vi "Position Mean - Plugin Main.vi"(11 "Shared Data from EMA":T2={"Impulse Positions"=[], "Parameter Impuls Series"=[], "Data File"={"Data Channels"=[], "Sample Rate"=0, "Channel List"=[]}, "desacc "={"Threshold 1 [Acc]"=7000.0, "Threshold 2 [% of TH1]"=60, "tolerance"=3, "Search WD "=0.1, " always use TH2"=FALSE, "Range"=2.0, "Max time"=120.0, "Min time"=20.0, "Velocity Threshold"=150}, "Experiment Parameters 2"={"Subject"="", "Strain"="", "Rotation plane"="", "Experimenter"="", "Trial"=0.0, "Time"=0.0}} {"Parameter Impuls Series"."Gain" format="%.1f"; "Parameter Impuls Series"."Offset" format="%.1f"}) -> (3 "Shared Data from EMA 2":T2={"Impulse Positions"=[], "Parameter Impuls Series"=[], "Data File"={"Data Channels"=[], "Sample Rate"=0, "Channel List"=[]}, "desacc "={"Threshold 1 [Acc]"=7000.0, "Threshold 2 [% of TH1]"=60, "tolerance"=3, "Search WD "=0.1, " always use TH2"=FALSE, "Range"=2.0, "Max time"=120.0, "Min time"=20.0, "Velocity Threshold"=150}, "Experiment Parameters 2"={"Subject"="", "Strain"="", "Rotation plane"="", "Experimenter"="", "Trial"=0.0, "Time"=0.0}} {"Parameter Impuls Series"."Gain" format="%.1f"; "Parameter Impuls Series"."Offset" format="%.1f"})   [LabVIEW 2013]
uses:
  Plugin Shared Data.ctl
  core/type-defs/TD_Impulse Parameter.ctl
  res/controls/impuls graph/impuls graph.xctl
  <vilib>/Analysis/baseanly.llb/Mean (DBL).vi
  comm/impulse/impulse functions.lvlib
  <vilib>/Analysis/NI_AALBase.lvlib
  <vilib>/ptbypt/NI_PtbyPt.lvlib
  core/core.lvlib
  plugin data.lvlib
panel:
  out "Waveform Graph":dbl[][](graph)
  out "Impulse Plot":T1(xcontrol)
  out "Waveform Graph 2":dbl[][](graph)
  in  "Delete trace":bool
  in  "Button toClipboard":bool
  in  "Button Save":bool
  in  "Table":string[][](table)
  out "K":dbl format="%#.3e"
  out "Distance":dbl format="%#.2g"
  out "Distance SD":dbl format="%#.2g"
  in  "Button Calculate":bool
  out "K SD":dbl format="%#.2g"
  in  "Parameter Impuls Series":T3=[{"Color"=4652800, "Visible"=TRUE, "Channel"=5, "Invert"=FALSE, "Desaccade"=FALSE, "Offset"=0.0, "Gain"=1.0}, {"Color"=16860, "Visible"=TRUE, "Channel"=13, "Invert"=FALSE, "Desaccade"=FALSE, "Offset"=0.0, "Gain"=1.0}, {"Color"=16711680, "Visible"=TRUE, "Channel"=21, "Invert"=FALSE, "Desaccade"=FALSE, "Offset"=0.0, "Gain"=1.0}] {"Gain" format="%.1f"; "Offset" format="%.1f"}
  in  "Impulse Direction":bool
  in  "Mean and STD":bool
  in  "Delete trace 2":bool
  in  "Stop Button":bool
  # "Offset         Gain    Inv                    Channel                         Col   Vis   Sac"
  # "Pos"
  # "Neg"
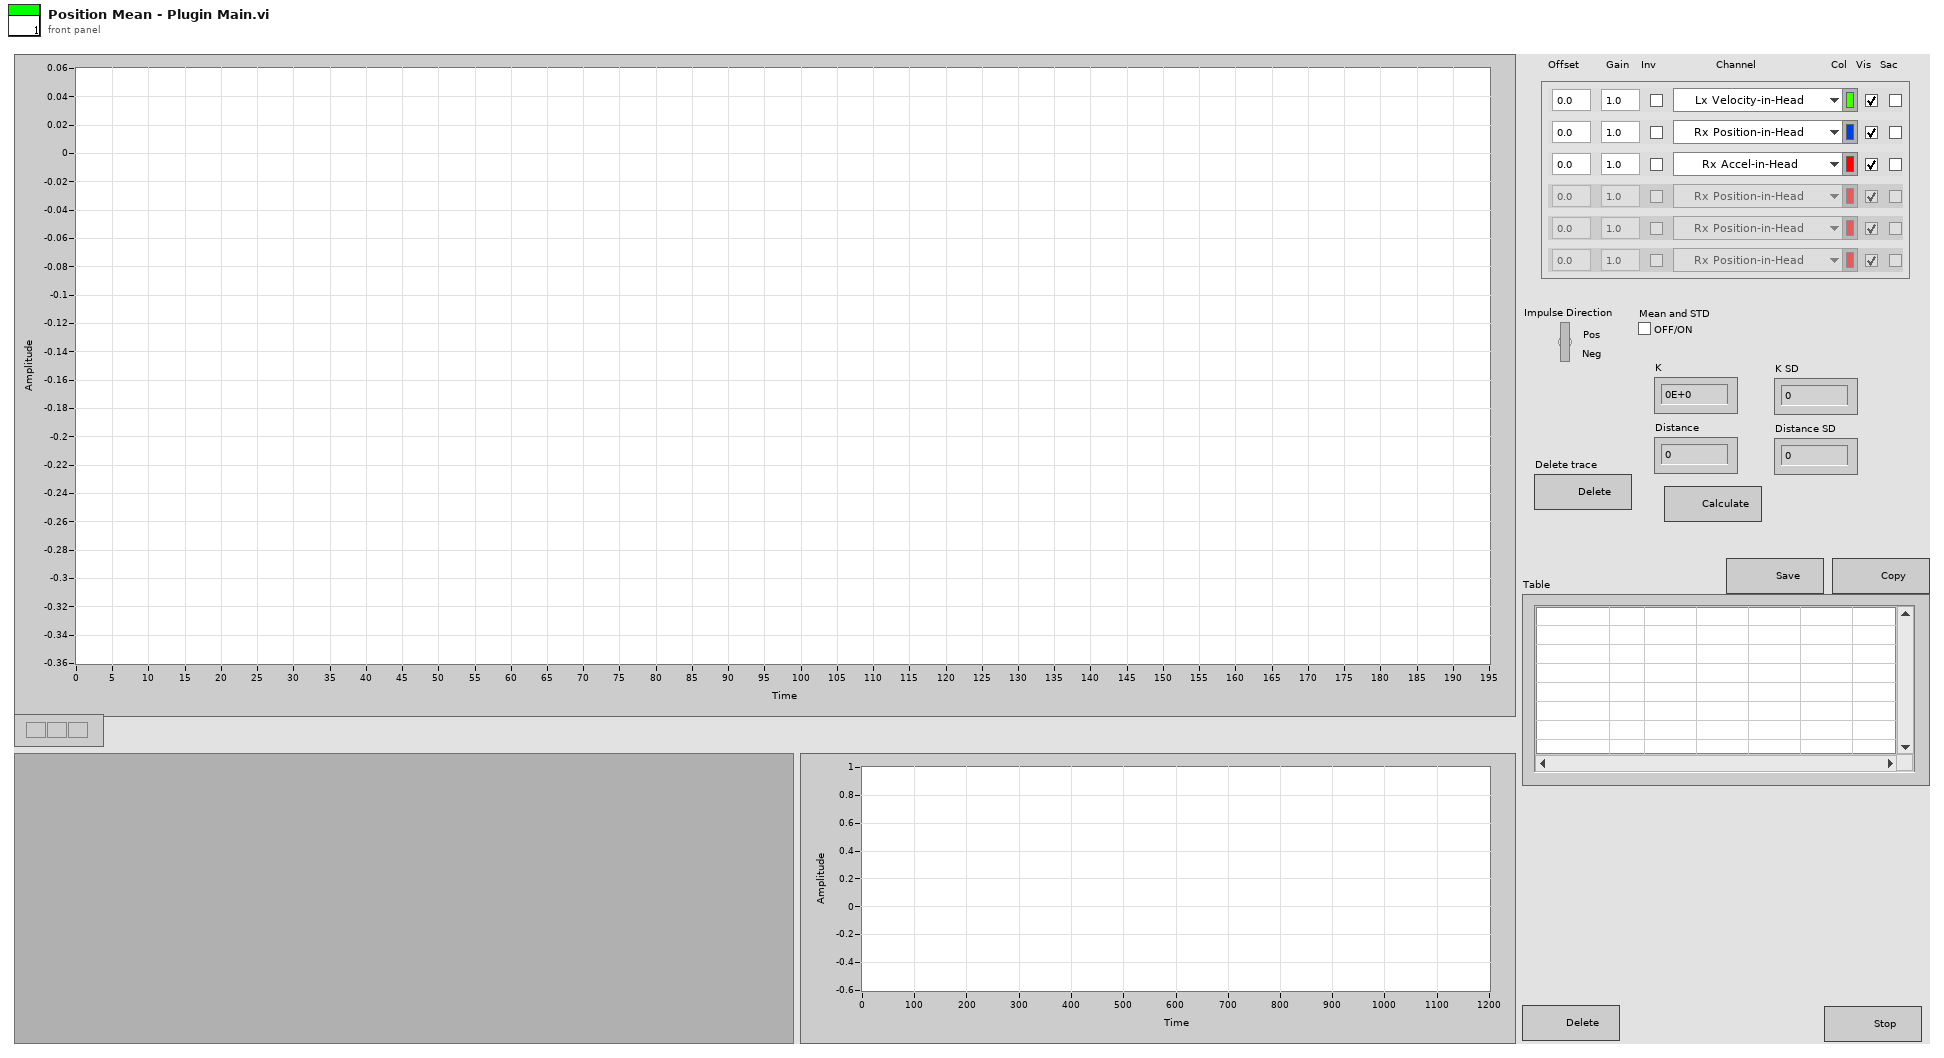
[diagram p1: front panel]
types:
  T1 = cluster{"Data":dbl[][], "Colour":u32, "Channel Name":string, "Sample Rate":dbl, "Visible":bool}[]
  T2 = typedef "plugin data.lvlib/Plugin Shared Data.ctl" = cluster{"Impulse Positions":cluster{"Start":i32, "End":i32, "Impulse Plane":enum16{"Other", "Yaw", "Pitch", "Roll", "LARP", "RALP"}, "Impulse Direction +ve?":bool, "Time offset":i32, "Amplitude offset":dbl}[], "Parameter Impuls Series":T3, "Data File":cluster{"Data Channels":dbl[][], "Sample Rate":i32, "Channel List":string[]}, "desacc ":cluster{"Threshold 1 [Acc]":dbl, "Threshold 2 [% of TH1]":i32, "tolerance":i32, "Search WD ":dbl, " always use TH2":bool, "Range":dbl, "Max time":dbl, "Min time":dbl, "Velocity Threshold":i32}, "Experiment Parameters 2":cluster{"Subject":string, "Strain":string, "Rotation plane":string, "Experimenter":string, "Trial":dbl, "Time":dbl}}
  T3 = typedef "core.lvlib/TD_Impulse Parameter.ctl" = cluster{"Color":u32, "Visible":bool, "Channel":u16, "Invert":bool, "Desaccade":bool, "Offset":dbl, "Gain":dbl}[]
  T4 = cluster{"Example Data":bool, "Impuls Data":cluster{"Data":dbl[][], "Colour":u32, "Channel Name":string, "Sample Rate":dbl, "Visible":bool}[], "K":dbl[], "cum pos data":dbl[][]}
  T5 = enum16{"Other", "Yaw", "Pitch", "Roll", "LARP", "RALP"}
  T6 = cluster{"Data Channels":dbl[][], "Sample Rate":i32, "Channel List":string[]}
  T7 = cluster{"Start":i32, "End":i32, "Impulse Plane":enum16{"Other", "Yaw", "Pitch", "Roll", "LARP", "RALP"}, "Impulse Direction +ve?":bool, "Time offset":i32, "Amplitude offset":dbl}[]
  T8 = cluster{"Threshold 1 [Acc]":dbl, "Threshold 2 [% of TH1]":i32, "tolerance":i32, "Search WD ":dbl, " always use TH2":bool, "Range":dbl, "Max time":dbl, "Min time":dbl, "Velocity Threshold":i32}
  T9 = typedef "LVCursorListTypeDef.ctl" = cluster{"Name":string, "Color":u32, "Style":u8, "Point Style":u8, "Name Visible":bool, "Allow Drag":bool, "Cursor Mode":u32, "Plot":i32, "Index":i32, "Position":cluster{"X":dbl, "Y":dbl}, "X Scale":u32, "Y Scale":u32, "Watch Plots":i32[], "Watch All Plots":bool, "Plot Area":i32, "Label Offset":cluster{"X":dbl, "Y":dbl}}[]
  T10 = cluster{"Name":string, "Color":u32, "Style":u8, "Point Style":u8, "Name Visible":bool, "Allow Drag":bool, "Cursor Mode":u32, "Plot":i32, "Index":i32, "Position":cluster{"X":dbl, "Y":dbl}, "X Scale":u32, "Y Scale":u32, "Watch Plots":i32[], "Watch All Plots":bool, "Plot Area":i32, "Label Offset":cluster{"X":dbl, "Y":dbl}}
  T11 = cluster{"Data":dbl[][], "Colour":u32, "Channel Name":string, "Sample Rate":dbl, "Visible":bool}
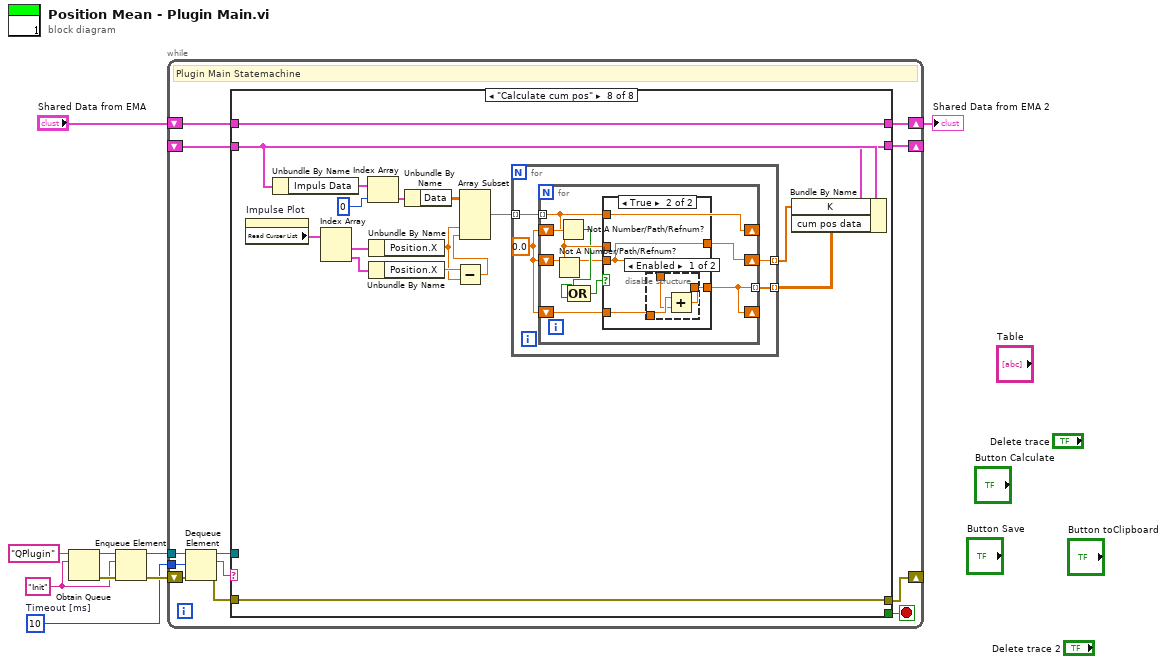
[diagram p0: block diagram]
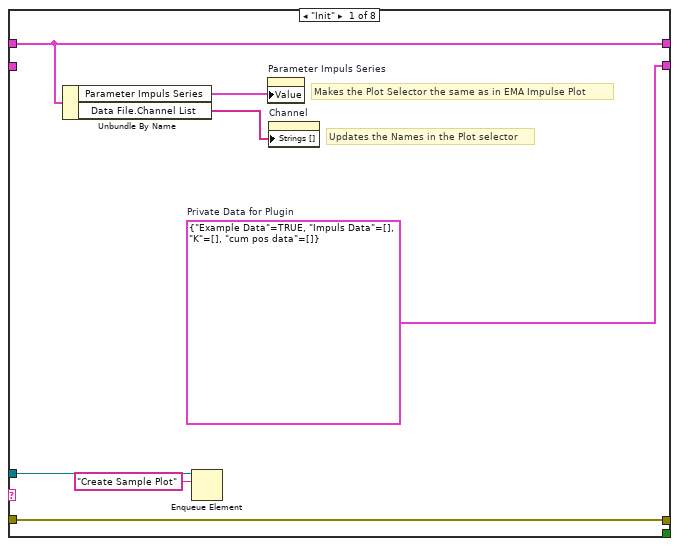
[diagram p2: hidden frame]
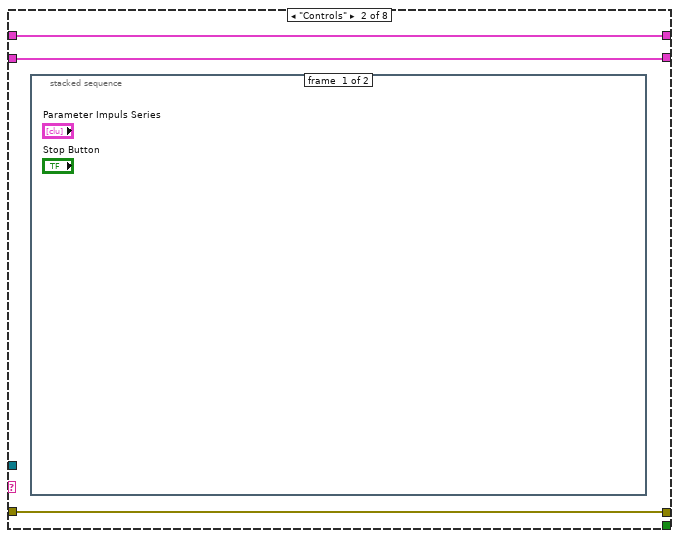
[diagram p3: hidden frame]
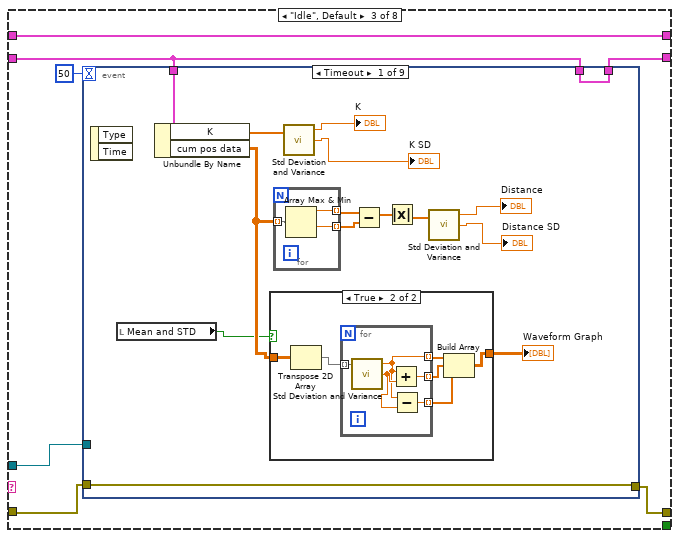
[diagram p5: hidden frame]
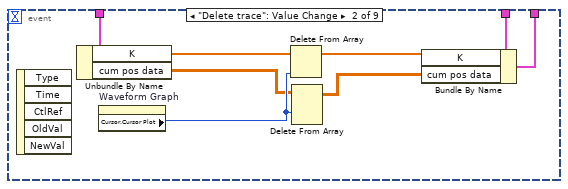
[diagram p7: hidden frame]
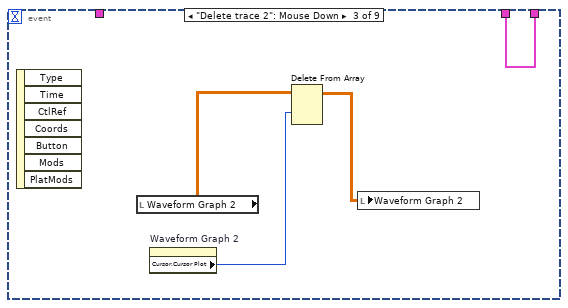
[diagram p8: hidden frame]
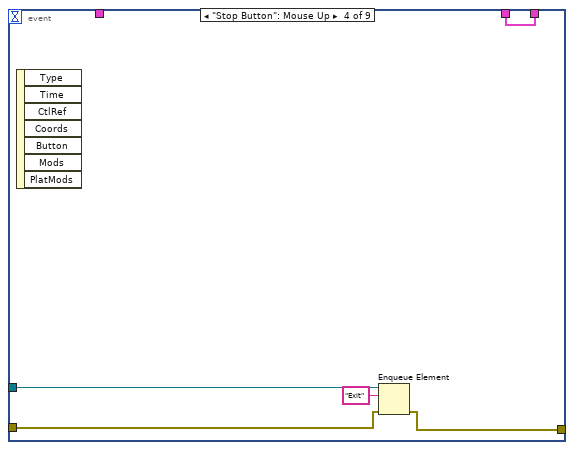
[diagram p9: hidden frame]
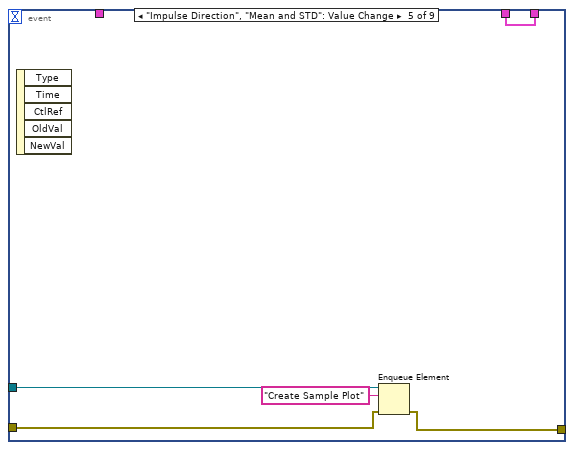
[diagram p10: hidden frame]
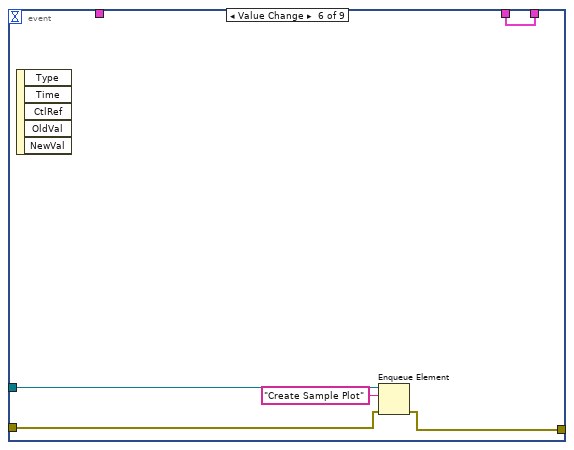
[diagram p11: hidden frame]
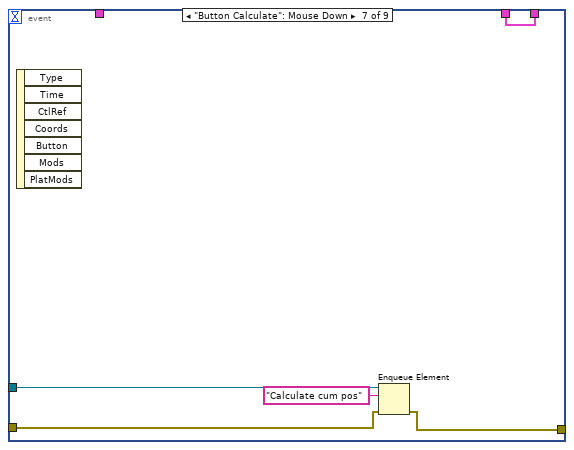
[diagram p12: hidden frame]
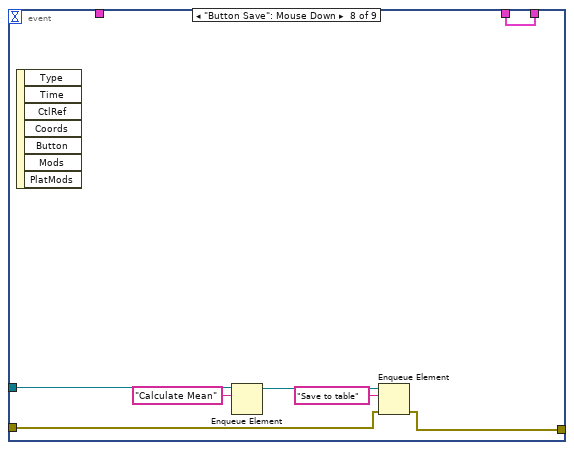
[diagram p13: hidden frame]
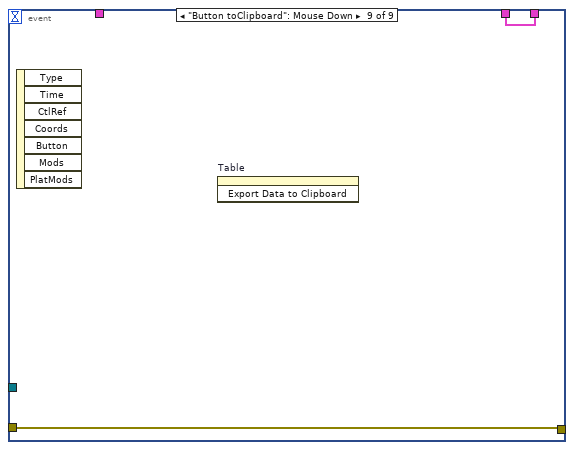
[diagram p14: hidden frame]
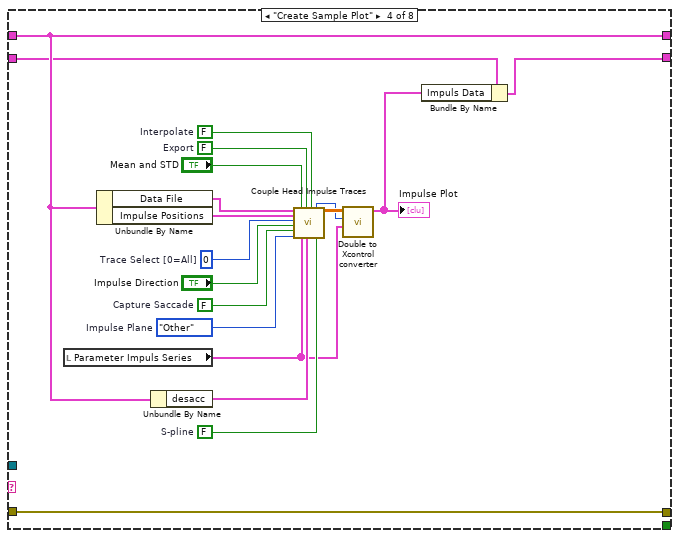
[diagram p15: hidden frame]
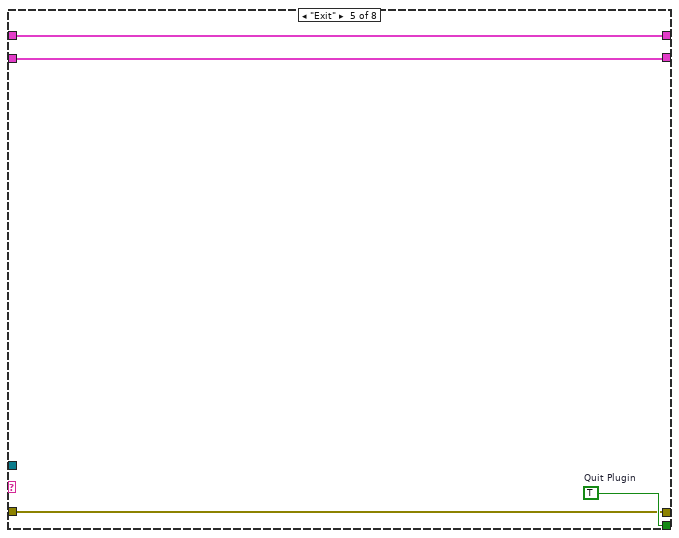
[diagram p16: hidden frame]
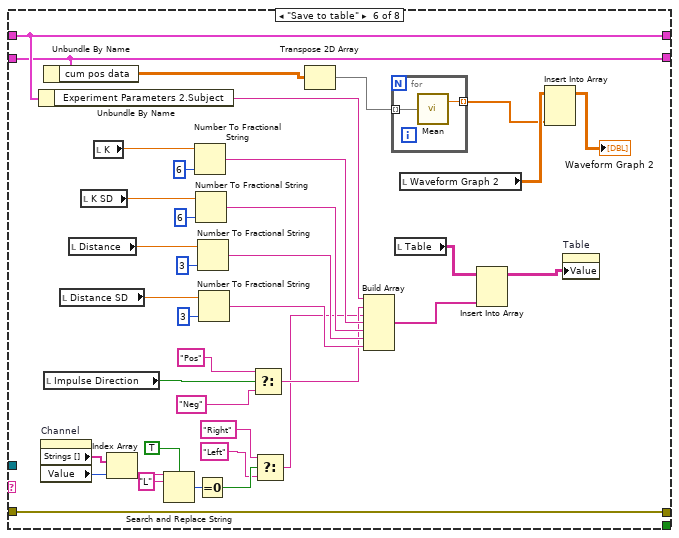
[diagram p17: hidden frame]
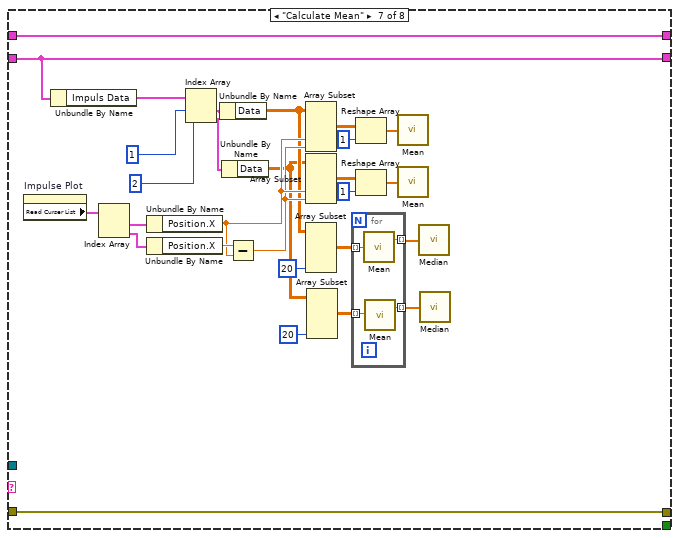
[diagram p18: hidden frame]
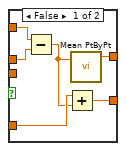
[diagram p19: hidden frame]
diagram:
  w3 = 10  # Timeout [ms]
  w7 = "Init"
  n1 = Obtain Queue(name (unnamed)="QPlugin", element data type=w7) -> (queue out=w8:refnum<queue>, error out=w9:errorcluster)  [unwired: 3 in, 1 out]
  n2 = Enqueue Element(queue=w8, element=w7, error in (no error)=w9) -> (queue out=w5:refnum<queue>, error out=w4:errorcluster)  [unwired: 1 in, 1 out]
  n3 = while {
    tunnel: w5 -> [w20]
    tunnel: w3 -> [w18]
    shift-right: [w14] -> _
    shift-left: w4 -> [w19]
    shift-right: [w13] -> _
    shift-left: _ -> [w12]
    shift-right: [w10] -> w1
    shift-left: "Shared Data from EMA" -> [w11]
    stop <- w21 stop-if-true
    # "Plugin Main Statemachine"
    n4 = Dequeue Element(queue=w20, timeout in ms (-1)=w18, error in (no error)=w19) -> (queue out=w17:refnum<queue>, element=w16:string, error out=w15:errorcluster)  [unwired: 1 out]
    n5 = case shown="\"Calculate cum pos\"" w16 {
      tunnel: [_ _ _ _ w132 _ _ _] -> w21
      tunnel: w17 -> [w26 _ w37 _ _ _ _ _]
      tunnel: w15 -> [w27 w29 w36 w128 w131 w170 w200 w221]
      tunnel: [w27 w29 w35 w128 w131 w170 w200 w221] -> w14
      tunnel: [w28 w30 w32 w111 w130 w138 w198 w207] -> w13
      tunnel: w12 -> [_ w30 w33 w112 w130 w138 w198 w208]
      tunnel: w11 -> [w24 w31 w38 w118 w129 w169 w199 w220]
      tunnel: [w24 w31 w38 w118 w129 w169 w199 w220] -> w10
      frame "Init" {
        w28 = T4 {"Example Data"=TRUE, "Impuls Data"=[], "K"=[], "cum pos data"=[]}  # Private Data for Plugin
        # "Makes the Plot Selector the same as in EMA Impulse Plot"
        # "Updates the Names in the Plot selector"
        n6 = Unbundle By Name(w24) -> ("Parameter Impuls Series"=w23:T3, "Data File.Channel List"=w22:string[])
        n7 = Enqueue Element(queue=w26, element="Create Sample Plot") -> ()  [unwired: 2 in, 3 out]
        n8 = property on="Parameter Impuls Series" class="Arr (strict)"("Value"=w23) -> ()  [unwired: 2 in, 2 out]
        n9 = property on="Channel" class="Ring (strict)"("Strings []"=w22) -> ()  [unwired: 2 in, 2 out]
      }
      frame "Controls" {
        n10 = stacked-sequence {
          frame #0 {
          }
          frame #1 {
          }
        }
      }
      frame "Idle", Default {
        n11 = event shown="[0] Timeout" {
          selector: _ -> [_ _ _ _ _ _ _ _ _]
          dyn-events: _ -> [_ _ _ _ _ _ _ _ _]
          timeout: 50 -> [_ _ _ _ _ _ _ _ _]
          tunnel: w37 -> [_ _ _ w85 w90 w95 w100 w104 _]
          tunnel: w36 -> [w53 _ _ w83 w88 w93 w98 w106 w109]
          tunnel: [w53 _ _ w82 w87 w92 w97 w105 w109] -> w35
          tunnel: w33 -> [w52 w76 _ _ _ _ _ _ _]
          tunnel: w33 -> [w51 w74 w80 w81 w86 w91 w96 w101 w108]
          tunnel: [w51 w71 w80 w81 w86 w91 w96 w101 w108] -> w32
          event Timeout {
            n12 = event-data() -> ()  [unwired: 1 in, 2 out]
            n13 = local read "Mean and STD"() -> (w45:bool)
            n14 = Unbundle By Name(w52) -> ("K"=w39:dbl[], "cum pos data"=w47:dbl[][])
            n15 = case shown="True" w45 {
              tunnel: w47 -> [w54 w60]
              tunnel: [w54 w57] -> w46
              frame False {
              }
              frame True {
                n16 = Transpose 2D Array(2D array=w60) -> (transposed array=w59:dbl[][])
                n17 = for {
                  tunnel: w59 -> [w65] mode=indexing
                  tunnel: [w61] -> w58 mode=indexing
                  tunnel: [w63] -> w56 mode=indexing
                  tunnel: [w62] -> w55 mode=indexing
                  n18 = call <vilib>:"Std Deviation and Variance.vi"("X"=w65) -> ("mean"=w61:dbl, "standard deviation"=w64:dbl)  [unwired: 1 in, 1 out]
                  n19 = Add(x=w61, y=w64) -> (x+y=w63:dbl)
                  n20 = Subtract(x=w61, y=w64) -> (x-y=w62:dbl)
                }
                n21 = Build Array(w58, w56, w55) -> (w57:dbl[][])
              }
            }
            "Waveform Graph" <- w46
            n22 = for {
              tunnel: w47 -> [w68] mode=indexing
              tunnel: [w67] -> w50 mode=indexing
              tunnel: [w66] -> w49 mode=indexing
              n23 = Array Max & Min(array=w68) -> (max value=w67:dbl, min value=w66:dbl)  [unwired: 2 out]
            }
            n24 = call <vilib>:"Std Deviation and Variance.vi"("X"=w39) -> ("mean"=→"K":dbl, "standard deviation"=→"K SD":dbl)  [unwired: 1 in, 1 out]
            n25 = Subtract(x=w50, y=w49) -> (x-y=w48:dbl[])
            n26 = Absolute Value(x=w48) -> (abs(x)=w44:dbl[])
            n27 = call <vilib>:"Std Deviation and Variance.vi"("X"=w44) -> ("mean"=→"Distance":dbl, "standard deviation"=→"Distance SD":dbl)  [unwired: 1 in, 1 out]
          }
          event "Delete trace": Value Change {
            n28 = event-data() -> ()  [unwired: 1 in, 5 out]
            n29 = Unbundle By Name(w76) -> ("K"=w75:dbl[], "cum pos data"=w69:dbl[][])
            n30 = property on="Waveform Graph" class="WFGraph (strict)"() -> ("Cursor.Cursor Plot"=w70:i32)  [unwired: 2 in, 2 out]
            n31 = Delete From Array(array=w75, index=w70) -> (array with subset deleted=w73:dbl[])  [unwired: 1 in, 1 out]
            n32 = Delete From Array(array=w69, index (row)=w70) -> (array with subset deleted=w72:dbl[][])  [unwired: 2 in, 1 out]
            n33 = Bundle By Name(cluster=w74, "K"=w73, "cum pos data"=w72) -> (w71:T4)
          }
          event "Delete trace 2": Mouse Down {
            n34 = event-data() -> ()  [unwired: 1 in, 7 out]
            n35 = local read "Waveform Graph 2"() -> (w79:dbl[][])
            n36 = property on="Waveform Graph 2" class="WFGraph (strict)"() -> ("Cursor.Cursor Plot"=w77:i32)  [unwired: 2 in, 2 out]
            n37 = Delete From Array(array=w79, index (row)=w77) -> (array with subset deleted=w78:dbl[][])  [unwired: 2 in, 1 out]
            n38 = local write "Waveform Graph 2"(w78) -> ()
          }
          event "Stop Button": Mouse Up {
            n39 = event-data() -> ()  [unwired: 1 in, 7 out]
            n40 = Enqueue Element(queue=w85, element="Exit", error in (no error)=w83) -> (error out=w82:errorcluster)  [unwired: 1 in, 2 out]
          }
          event "Impulse Direction", "Mean and STD": Value Change {
            n41 = event-data() -> ()  [unwired: 1 in, 5 out]
            n42 = Enqueue Element(queue=w90, element="Create Sample Plot", error in (no error)=w88) -> (error out=w87:errorcluster)  [unwired: 1 in, 2 out]
          }
          event Value Change {
            n43 = event-data() -> ()  [unwired: 1 in, 5 out]
            n44 = Enqueue Element(queue=w95, element="Create Sample Plot", error in (no error)=w93) -> (error out=w92:errorcluster)  [unwired: 1 in, 2 out]
          }
          event "Button Calculate": Mouse Down {
            n45 = event-data() -> ()  [unwired: 1 in, 7 out]
            n46 = Enqueue Element(queue=w100, element="Calculate cum pos", error in (no error)=w98) -> (error out=w97:errorcluster)  [unwired: 1 in, 2 out]
          }
          event "Button Save": Mouse Down {
            n47 = event-data() -> ()  [unwired: 1 in, 7 out]
            n48 = Enqueue Element(queue=w104, element="Calculate Mean") -> (queue out=w103:refnum<queue>)  [unwired: 2 in, 2 out]
            n49 = Enqueue Element(queue=w103, element="Save to table", error in (no error)=w106) -> (error out=w105:errorcluster)  [unwired: 1 in, 2 out]
          }
          event "Button toClipboard": Mouse Down {
            n50 = event-data() -> ()  [unwired: 1 in, 7 out]
            n51 = invoke on="Table" class="Tbl (strict)" method="Export Data to Clipboard"() -> ()  [unwired: 3 in, 3 out]
          }
        }
      }
      frame "Create Sample Plot" {
        w116 = FALSE  # S-pline
        w119 = FALSE  # Interpolate
        w120 = FALSE  # Export
        w122 = T5."Other"  # Impulse Plane
        w123 = FALSE  # Capture Saccade
        w125 = 0  # Trace Select [0=All]
        n52 = local read "Parameter Impuls Series"() -> (w113:T3)
        n53 = Unbundle By Name(w118) -> ("Data File"=w126:T6, "Impulse Positions"=w127:T7)
        n54 = Unbundle By Name(w118) -> ("desacc"=w117:T8)
        n55 = call "Couple Head Impulse Traces.vi"("Data Input"=w126, "Impulse Positions"=w127, "Trace Select"=w125, "Impulse Direction +ve?"="Impulse Direction", "Capture Saccade"=w123, "Impulse Plane"=w122, "Mean and STD"="Mean and STD", "Plot Selection 2"=w113, "Export"=w120, "desacc"=w117, "Interpolate"=w119, "S-pline"=w116) -> ("No Impulses"=w114:i32, "Impulses"=w115:dbl[][])  [unwired: 4 in, 2 out]
        n56 = call "Double to Xcontrol converter.vi"("Parameter Impuls Series"=w113, "No Impulses"=w114, "Impulses"=w115) -> ("Array"=w110:T1)  [unwired: 8 in]
        "Impulse Plot" <- w110
        n57 = Bundle By Name(cluster=w112, "Impuls Data"=w110) -> (w111:T4)
      }
      frame "Exit" {
        w132 = TRUE  # Quit Plugin
      }
      frame "Save to table" {
        n58 = Unbundle By Name(w169) -> ("Experiment Parameters 2.Subject"=w167:string)
        n59 = property on="Channel" class="Ring (strict)"() -> ("Strings []"=w148:string[], "Value"=w147:u16)  [unwired: 2 in, 2 out]
        n60 = Unbundle By Name(w138) -> ("cum pos data"=w136:dbl[][])
        n61 = local read "Impulse Direction"() -> (w152:bool)
        n62 = local read "Distance SD"() -> (w157:dbl)
        n63 = local read "Distance"() -> (w158:dbl)
        n64 = local read "K SD"() -> (w159:dbl)
        n65 = local read "K"() -> (w166:dbl)
        n66 = Index Array(array=w148, index=w147) -> (element=w146:string)
        n67 = Search and Replace String(case sensitive?=TRUE ("ignore case? (F)"), input string=w146, search string="L") -> (number of replacements=w143:i32)  [unwired: 5 in, 3 out]
        n68 = Number To Fractional String(number=w166, precision (6)=i16 6) -> (F-format string=w156:string)  [unwired: 2 in]
        n69 = Number To Fractional String(number=w159, precision (6)=i16 6) -> (F-format string=w155:string)  [unwired: 2 in]
        n70 = Equal To 0?(x=w143) -> (x = 0?=w142:bool)
        n71 = Number To Fractional String(number=w158, precision (6)=i16 3) -> (F-format string=w154:string)  [unwired: 2 in]
        n72 = Number To Fractional String(number=w157, precision (6)=i16 3) -> (F-format string=w153:string)  [unwired: 2 in]
        n73 = Select(t="Pos", s=w152, f="Neg") -> (s? t:f=w151:string)
        n74 = Select(t="Right", s=w142, f="Left") -> (s? t:f=w139:string)
        n75 = Transpose 2D Array(2D array=w136) -> (transposed array=w137:dbl[][])
        n76 = Build Array(w167, w151, w139, w156, w155, w154, w153) -> (w164:string[])
        n77 = for {
          tunnel: w137 -> [w172] mode=indexing
          tunnel: [w171] -> w134 mode=indexing
          n78 = call-poly <vilib>:"Mean.vi"("X"=w172) -> ("mean"=w171:dbl)  [unwired: 1 out]
        }
        n79 = local read "Table"() -> (w168:string[][])
        n80 = local read "Waveform Graph 2"() -> (w135:dbl[][])
        n81 = Insert Into Array(array=w168, new element=w164) -> (w163:string[][])  [unwired: 2 in]
        n82 = Insert Into Array(array=w135, new element=w134) -> (→"Waveform Graph 2":dbl[][])  [unwired: 2 in]
        n83 = property on="Table" class="Tbl (strict)"("Value"=w163) -> ()  [unwired: 2 in, 2 out]
      }
      frame "Calculate Mean" {
        n84 = property on="Impulse Plot" class="impuls graph (strict)"() -> ("Read Curser List"=w194:T9)  [unwired: 2 in, 2 out]
        n85 = Unbundle By Name(w198) -> ("Impuls Data"=w197:T1)
        n86 = Index Array(array=w194) -> (element #1=w193:T10, element #2=w192:T10)  [unwired: 2 in]
        n87 = Unbundle By Name(w193) -> ("Position.X"=w182:dbl)
        n88 = Unbundle By Name(w192) -> ("Position.X"=w191:dbl)
        n89 = Index Array(array=w197, index #1=1 ("index"), index #2=2 ("index")) -> (element #1=w195:T11, element #2=w183:T11)
        n90 = Unbundle By Name(w195) -> ("Data"=w180:dbl[][])
        n91 = Unbundle By Name(w183) -> ("Data"=w179:dbl[][])
        n92 = Subtract(x=w191, y=w182) -> (x-y=w181:dbl)
        n93 = Array Subset(array=w180, index (col)=w182, length (col)=w181) -> (w190:dbl[][])  [unwired: 2 in]
        n94 = Array Subset(array=w179, index (col)=w182, length (col)=w181) -> (w184:dbl[][])  [unwired: 2 in]
        n95 = Array Subset(array=w180, length (col)=20 ("length")) -> (w176:dbl[][])  [unwired: 3 in]
        n96 = Array Subset(array=w179, length (col)=20 ("length")) -> (w175:dbl[][])  [unwired: 3 in]
        n97 = for {
          tunnel: w176 -> [w204] mode=indexing
          tunnel: w175 -> [w203] mode=indexing
          tunnel: [w202] -> w173 mode=indexing
          tunnel: [w201] -> w174 mode=indexing
          n98 = call-poly <vilib>:"Mean.vi"("X"=w204) -> ("mean"=w201:dbl)  [unwired: 1 out]
          n99 = call-poly <vilib>:"Mean.vi"("X"=w203) -> ("mean"=w202:dbl)  [unwired: 1 out]
        }
        n100 = Reshape Array(w190, 1 ("dimension size")) -> (w188:dbl[])
        n101 = Reshape Array(w184, 1 ("dimension size")) -> (w186:dbl[])
        n102 = call-poly <vilib>:"Mean.vi"("X"=w188) -> ()  [unwired: 2 out]
        n103 = call-poly <vilib>:"Mean.vi"("X"=w186) -> ()  [unwired: 2 out]
        n104 = call <vilib>:"Median.vi"("X"=w174) -> ()  [unwired: 2 out]
        n105 = call <vilib>:"Median.vi"("X"=w173) -> ()  [unwired: 2 out]
      }
      frame "Calculate cum pos" {
        n106 = property on="Impulse Plot" class="impuls graph (strict)"() -> ("Read Curser List"=w216:T9)  [unwired: 2 in, 2 out]
        n107 = Unbundle By Name(w208) -> ("Impuls Data"=w219:T1)
        n108 = Index Array(array=w216) -> (element #1=w215:T10, element #2=w214:T10)  [unwired: 2 in]
        n109 = Index Array(array=w219, index=0) -> (element=w217:T11)
        n110 = Unbundle By Name(w215) -> ("Position.X"=w211:dbl)
        n111 = Unbundle By Name(w214) -> ("Position.X"=w212:dbl)
        n112 = Unbundle By Name(w217) -> ("Data"=w213:dbl[][])
        n113 = Subtract(x=w212, y=w211) -> (x-y=w210:dbl)
        n114 = Array Subset(array=w213, index (col)=w211, length (col)=w210) -> (w209:dbl[][])  [unwired: 2 in]
        n115 = for {
          tunnel: w209 -> [w225] mode=indexing
          tunnel: [w224] -> w205 mode=indexing
          tunnel: [w222] -> w206 mode=indexing
          w223 = 0.0
          n116 = for {
            tunnel: w225 -> [w233] mode=indexing
            shift-right: [w233] -> _
            shift-left: w223 -> [w234]
            tunnel: [w228] -> w224 mode=indexing
            shift-right: [w228] -> _
            shift-left: w223 -> [w229]
            shift-right: [w227] -> w222
            shift-left: w223 -> [w226]
            n117 = Not A Number/Path/Refnum?(number/path/refnum=w234) -> (NaN/Path/Refnum?=w231:bool)
            n118 = Not A Number/Path/Refnum?(number/path/refnum=w233) -> (NaN/Path/Refnum?=w232:bool)
            n119 = Compound Arithmetic op=OR(w232, w231) -> (w230:bool)
            n120 = case shown="True" w230 {
              tunnel: w233 -> [w240 _]
              tunnel: w234 -> [w239 _]
              tunnel: [w238 w242] -> w228
              tunnel: w229 -> [w237 w243]
              tunnel: [w235 w241] -> w227
              tunnel: w226 -> [_ w241]
              frame False {
                n121 = Subtract(x=w240, y=w239) -> (x-y=w236:dbl)
                n122 = Add(x=w237, y=w236) -> (x+y=w238:dbl)
                n123 = call <vilib>:"Mean PtByPt.vi"("x"=w236) -> ("mean"=w235:dbl)  [unwired: 3 in, 1 out]
              }
              frame True {
                n124 = disable-structure shown="Enabled" {
                  disable-tunnel: w243 -> [w246 w247]
                  disable-tunnel: [w245 w247] -> w242
                  disable-tunnel: w241 -> [w244 _]
                  frame Enabled {
                    n125 = Add(x=w246, y=w244) -> (x+y=w245:dbl)
                  }
                  frame Disabled {
                  }
                }
              }
            }
          }
        }
        n126 = Bundle By Name(cluster=w208, "K"=w206, "cum pos data"=w205) -> (w207:T4)
      }
    }
  }
  "Shared Data from EMA 2" <- w1
